vi "Parseval Demo.vi"() -> ()   [LabVIEW 2015]
uses:
  <vilib>/Analysis/5stat.llb/RMS (DBL).vi
  Math VIs/FFT x(t) to dB,Degrees (1D).vi
  Math VIs/dB to Linear (1D).vi
  <vilib>/Analysis/NI_AALBase.lvlib
  <vilib>/Analysis/NI_AALPro.lvlib
panel:
  out "spec rss":dbl
  out "time ss":dbl
  out "spec rms":dbl format="%0.6f"
  out "time rms":dbl format="%0.6f"
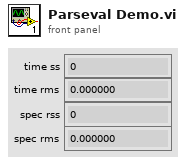
[diagram p1: front panel]
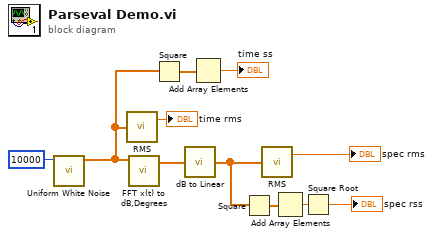
[diagram p0: block diagram]
diagram:
  n1 = call <vilib>:"Uniform White Noise.vi"("samples"=10000) -> ("uniform white noise"=w7:dbl[])  [unwired: 9 in, 1 out]
  n2 = call-poly <vilib>:"RMS.vi"("X"=w7) -> ("rms value"=→"time rms":dbl)  [unwired: 1 out]
  n3 = call-poly "FFT x(t) to dB,Degrees.vi"("X"=w7) -> ("+Freq. Mag of FFT (dB rms)"=w9:dbl[])  [unwired: 8 in, 2 out]
  n4 = Square(x=w7) -> (x^2=w6:dbl[])
  n5 = call-poly "dB to Linear.vi"("dB"=w9) -> ("linear"=w3:dbl[])
  n6 = Add Array Elements(numeric array=w6) -> (sum=→"time ss":dbl)
  n7 = Square(x=w3) -> (x^2=w4:dbl[])
  n8 = call-poly <vilib>:"RMS.vi"("X"=w3) -> ("rms value"=→"spec rms":dbl)  [unwired: 1 out]
  n9 = Add Array Elements(numeric array=w4) -> (sum=w2:dbl)
  n10 = Square Root(x=w2) -> (sqrt(x)=→"spec rss":dbl)
